vi "Render Recursive Partial without Recursion.vi"(8 "Error In":errorcluster) -> (0 "Error Out":errorcluster)   [LabVIEW 2018, in "Tests.lvlib" / "Render.lvlib"]
uses:
  Render.lvlib
  <vilib>/addons/_JKI Toolkits/Caraya/classes/Test/Test.lvclass
  <vilib>/addons/_JKI Toolkits/Caraya/classes/Assert/Assert.lvclass
  src/Toolkit/Low-Level/Loaders/String/String.lvclass
  src/Toolkit/Low-Level/Support/Lex String.vi
  src/Toolkit/Data/Map/Map.lvclass
  src/Toolkit/Low-Level/Renderer/Abstract/Render to String.vi
  src/Toolkit/Data/Map/Support/From String.vi
  src/Toolkit/Low-Level/Compiler/Compiler.lvclass
  D:/Users/cfield/Code/Field R&D Services/Labstache/src/Toolkit/Low-Level/Loaders/Loader/Loader.lvclass
  D:/Users/cfield/Code/Field R&D Services/Labstache/src/Toolkit/Data/Datum/Datum.lvclass
  src/Toolkit/Low-Level/Nodes/Root/Root.lvclass
  D:/Users/cfield/Code/Field R&D Services/Labstache/src/Toolkit/Low-Level/Nodes/NonTerminal/NonTerminal.lvclass
  D:/Users/cfield/Code/Field R&D Services/Labstache/src/Toolkit/Low-Level/Nodes/Node/Node.lvclass
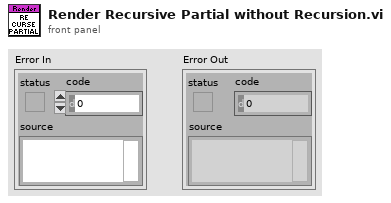
[diagram p1: front panel]
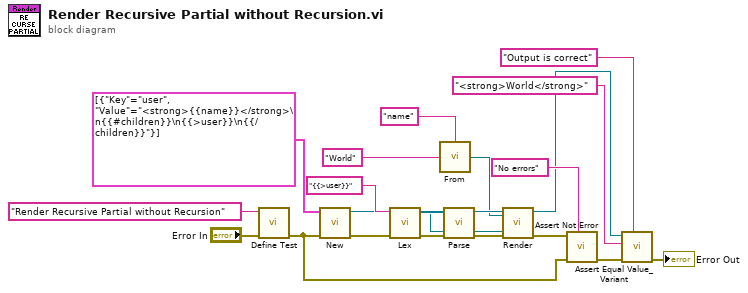
[diagram p0: block diagram]
diagram:
  n1 = call <vilib>:"Define Test.vi"("error in (no error)"="Error In", "Label (VI Title)"="Render Recursive Partial without Recursion") -> ("error out"=w7:errorcluster)  [unwired: 9 in]
  n2 = call "New.vi"("Error In"=w7, "Key-Value Pairs"=cluster{"Key":string, "Value":string}[] [{"Key"="user", "Value"="<strong>{{name}}</strong>\n{{#children}}\n{{>user}}\n{{/children}}"}]) -> ("Error Out"=w9:errorcluster, "String"=w4:refnum<class "String.lvclass">)  [unwired: 8 in]
  n3 = call-poly "Lex.vi"("Error In"=w9, "Input"="{{>user}}" ("format string")) -> ("Error Out"=w11:errorcluster, "Tokens"=w12:refnum<class "Token.lvclass">[])  [unwired: 8 in]
  n4 = call-poly "From.vi"("Value"="World", "Key"="name") -> ("Map"=w3:refnum<class "Map.lvclass">)
  n5 = call "Parse.vi"("Error In"=w11, "Tokens"=w12) -> ("Error Out"=w13:errorcluster, "Abstract Syntax Tree"=w10:refnum<class "Root.lvclass">)  [unwired: 8 in]
  n6 = call-poly "Render.vi"(6:w4, 7:w3, "Error In"=w13, "Context In"=w10) -> ("Error Out"=w15:errorcluster, "Context Out"=w14:refnum<class "Compiler.lvclass">)  [unwired: 5 in, 1 out]
  n7 = call <vilib>:"Assert Not Error.vi"("Label"="No errors", "error in (no error)"=w7, "Not Error?"=w15) -> ("error out"=w18:errorcluster)  [unwired: 8 in]
  n8 = call <vilib>:"Assert Equal Value_Variant.vi"("Label"="Output is correct", "error in (no error)"=w18, "Y"="<strong>World</strong>", "X"=w14) -> ("error out"=→"Error Out":errorcluster)  [unwired: 7 in]
